vi "CalcExpTotalTime.vi"(8 "error in (no error)":errorcluster, 10 "Current Temperature":dbl, 11 "RampProgramModel in":refnum<class "RampProgramModel.lvclass">) -> (0 "error out":errorcluster, 2 "TotalExpTime(sec)":dbl, 3 "RampProgramModel out":refnum<class "RampProgramModel.lvclass">)   [LabVIEW 2013, in "RampProgramModel.lvclass"]
uses:
  RampProgramModel.lvclass
  RampProgramModel.lvclass/RampProgramModel.ctl
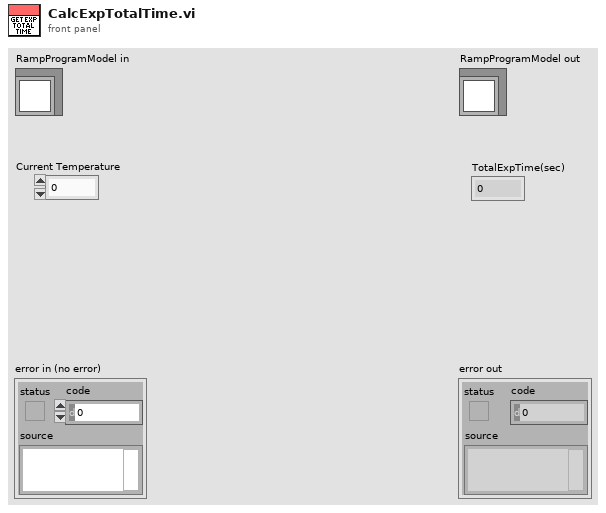
[diagram p1: front panel]
types:
  T1 = cluster{"SP (°C)":dbl, "Cooling rate (°C/min)":dbl, "Dwell Time @ SP (sec)":u32}[]
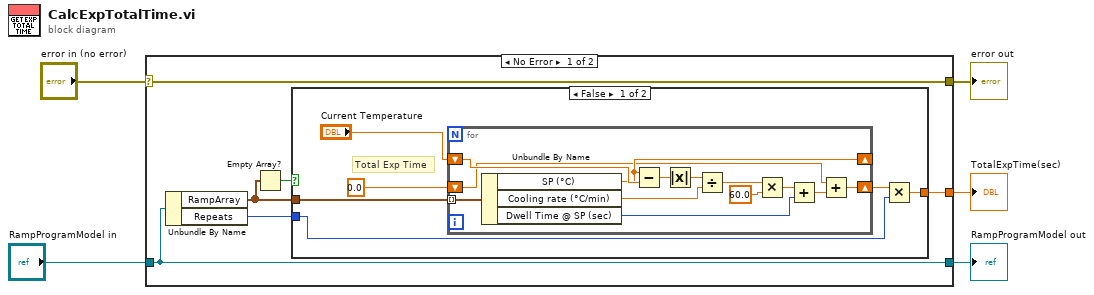
[diagram p0: block diagram]
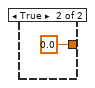
[diagram p2: hidden frame]
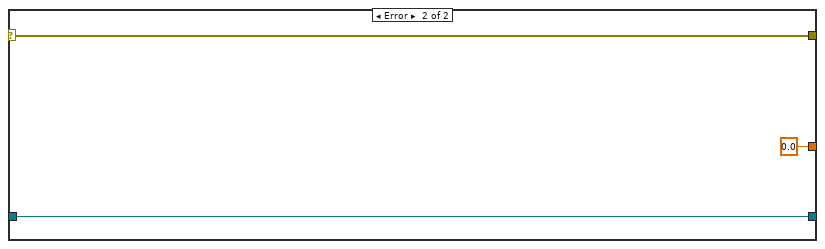
[diagram p3: hidden frame]
diagram:
  n1 = case shown="No Error" "error in (no error)" {
    selector: "error in (no error)" -> [w11 w34]
    tunnel: [w11 w34] -> w4
    tunnel: [w10 w33] -> w2
    tunnel: "RampProgramModel in" -> [w10 w33]
    tunnel: [w8 0.0 ("TotalExpTime(sec)")] -> w1
    frame No Error {
      n2 = Unbundle By Name(w10) -> ("RampArray"=w7:T1, "Repeats"=w6:u32)
      n3 = Empty Array?(array=w7) -> (empty?=w9:bool)
      n4 = case shown="False" w9 {
        tunnel: [w12 0.0 ("TotalExpTime(sec)")] -> w8
        tunnel: w7 -> [w17 _]
        tunnel: w6 -> [w13 _]
        frame False {
          # "Total Exp Time"
          n5 = for {
            tunnel: w17 -> [w30] mode=indexing
            shift-right: [w21] -> _
            shift-left: "Current Temperature" -> [w29]
            shift-right: [w18] -> w14
            shift-left: 0.0 -> [w20]
            n6 = Unbundle By Name(w30) -> ("SP (°C)"=w21:dbl, "Cooling rate (°C/min)"=w26:dbl, "Dwell Time @ SP (sec)"=w22:u32)
            n7 = Subtract(x=w21, y=w29) -> (x-y=w28:dbl)
            n8 = Absolute Value(x=w28) -> (abs(x)=w27:dbl)
            n9 = Divide(x=w27, y=w26) -> (x/y=w25:dbl)
            n10 = Multiply(x=w25, y=60.0) -> (x*y=w23:dbl)
            n11 = Add(x=w23, y=w22) -> (x+y=w19:dbl)
            n12 = Add(x=w20, y=w19) -> (x+y=w18:dbl)
          }
          n13 = Multiply(x=w14, y=w13) -> (x*y=w12:dbl)
        }
        frame True {
        }
      }
    }
    frame Error {
    }
  }
  "error out" <- w4
  "RampProgramModel out" <- w2
  "TotalExpTime(sec)" <- w1
